vi "flow meter test 2.vi"() -> ()   [LabVIEW 2013]
uses:
  <vilib>/Platform/TimedLoop/XDataNode/timing_clust.ctl
  <vilib>/Platform/TimedLoop/XDataNode/nitl_modes.ctl
  <vilib>/Platform/TimedLoop/XDataNode/wakeup.ctl
  <vilib>/rvi/FXPMathLib/FxpDiv/subVIs/nifxpmath_Div_SimConfig.ctl
  <vilib>/rvi/Emulation/niFpgaSctlEmulationGetInTimedLoop.vi
  <vilib>/rvi/Emulation/niFpgaEmulationReportErrorSimple.vi
  <vilib>/rvi/Emulation/niFpgaGetClockAttributes.vi
  ADC AI Global.vi
  <vilib>/rvi/Emulation/niFpgaProcessEmulError.vi
  ADC AI Global (Avg).vi
  <vilib>/rvi/Emulation/niFpgaCriticalErrorInLSC.vi
  <vilib>/rvi/eio/common/nirviEmuTemplateMethod_errors.vi
  <vilib>/rvi/FXPMathLib/FxpDiv/simVIs/DllFxpDivTemp_sub.vi
  <vilib>/Platform/TimedLoop/XDataNode/XDataNode.xnode
  <vilib>/eio/EIONode/EIONode.xnode
  <vilib>/rvi/FXPMathLib/FxpDiv/XNode/nifxpmath_Div.xnode
  <vilib>/Platform/TimedLoop/XDataNode/XDNodeRunTimeDep.lvlib
panel:
  out "Array 2":fxp<+/-,28,17>[](array[numeric])
  out "Array":fxp<+/-,28,17>[](array[numeric])
  out "Flow":fxp<+/-,28,17>[](array[numeric])
  in  "Freq Flow?":bool
  in  "Max Period (ticks)":u32
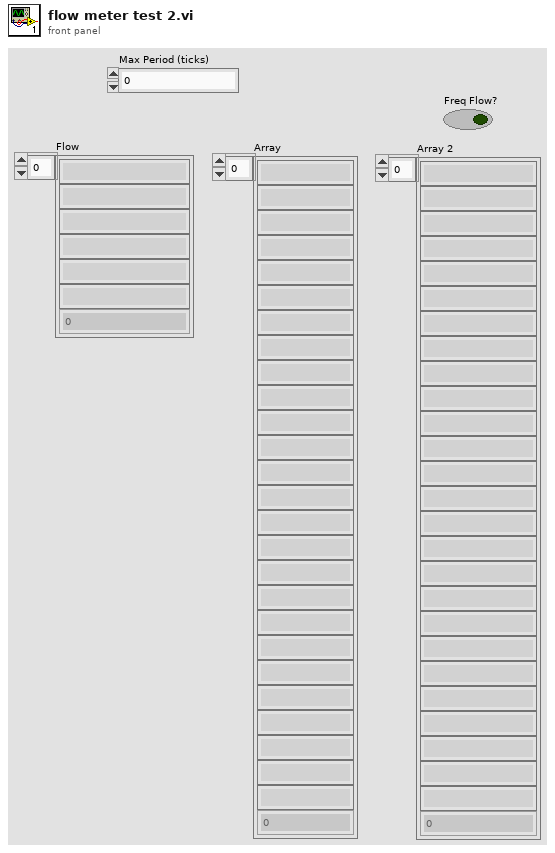
[diagram p1: front panel]
types:
  T1 = typedef "XDNodeRunTimeDep.lvlib/timing_clust.ctl" = cluster{"Expected End [f-1]":u64, "Actual End [f-1]":u64, "Finished Late? [f-1]":bool, "Expected End [i-1]":u64, "Actual End [i-1]":u64, "Finished Late? [i-1]":bool, "Expected Start [i]":u64, "Actual Start [i]":u64, "Expected Start [f]":u64, "Actual Start [f]":u64, "Source Name":string, "Structure Name":string, "Period":i64, "Deadline":i64, "Offset":i64, "Start":i64, "Priority":i32, "Timeout":i32, "Mode":T2, "Wakeup Reason":T3, "Error":errorcluster, "Source Type":string, "Secondary Source Type":string, "Global End Time":u64, "Global Start Time":u64, "Frame Duration":u64, "Iteration Duration":u64, "Assigned CPU":i32, "I/O Scan Engine Mode":u32}
  T2 = typedef "XDNodeRunTimeDep.lvlib/nitl_modes.ctl" = enum32{"No Change", "Process missed periods, maintain original phase", "Discard missed periods, maintain original phase", "Process missed periods, ignore original phase", "Discard missed periods, ignore original phase"}
  T3 = typedef "XDNodeRunTimeDep.lvlib/wakeup.ctl" = enum32{"Normal", "Aborted", "Asynchronous wakeup", "Timing source error", "Timed loop error", "Timeout"}
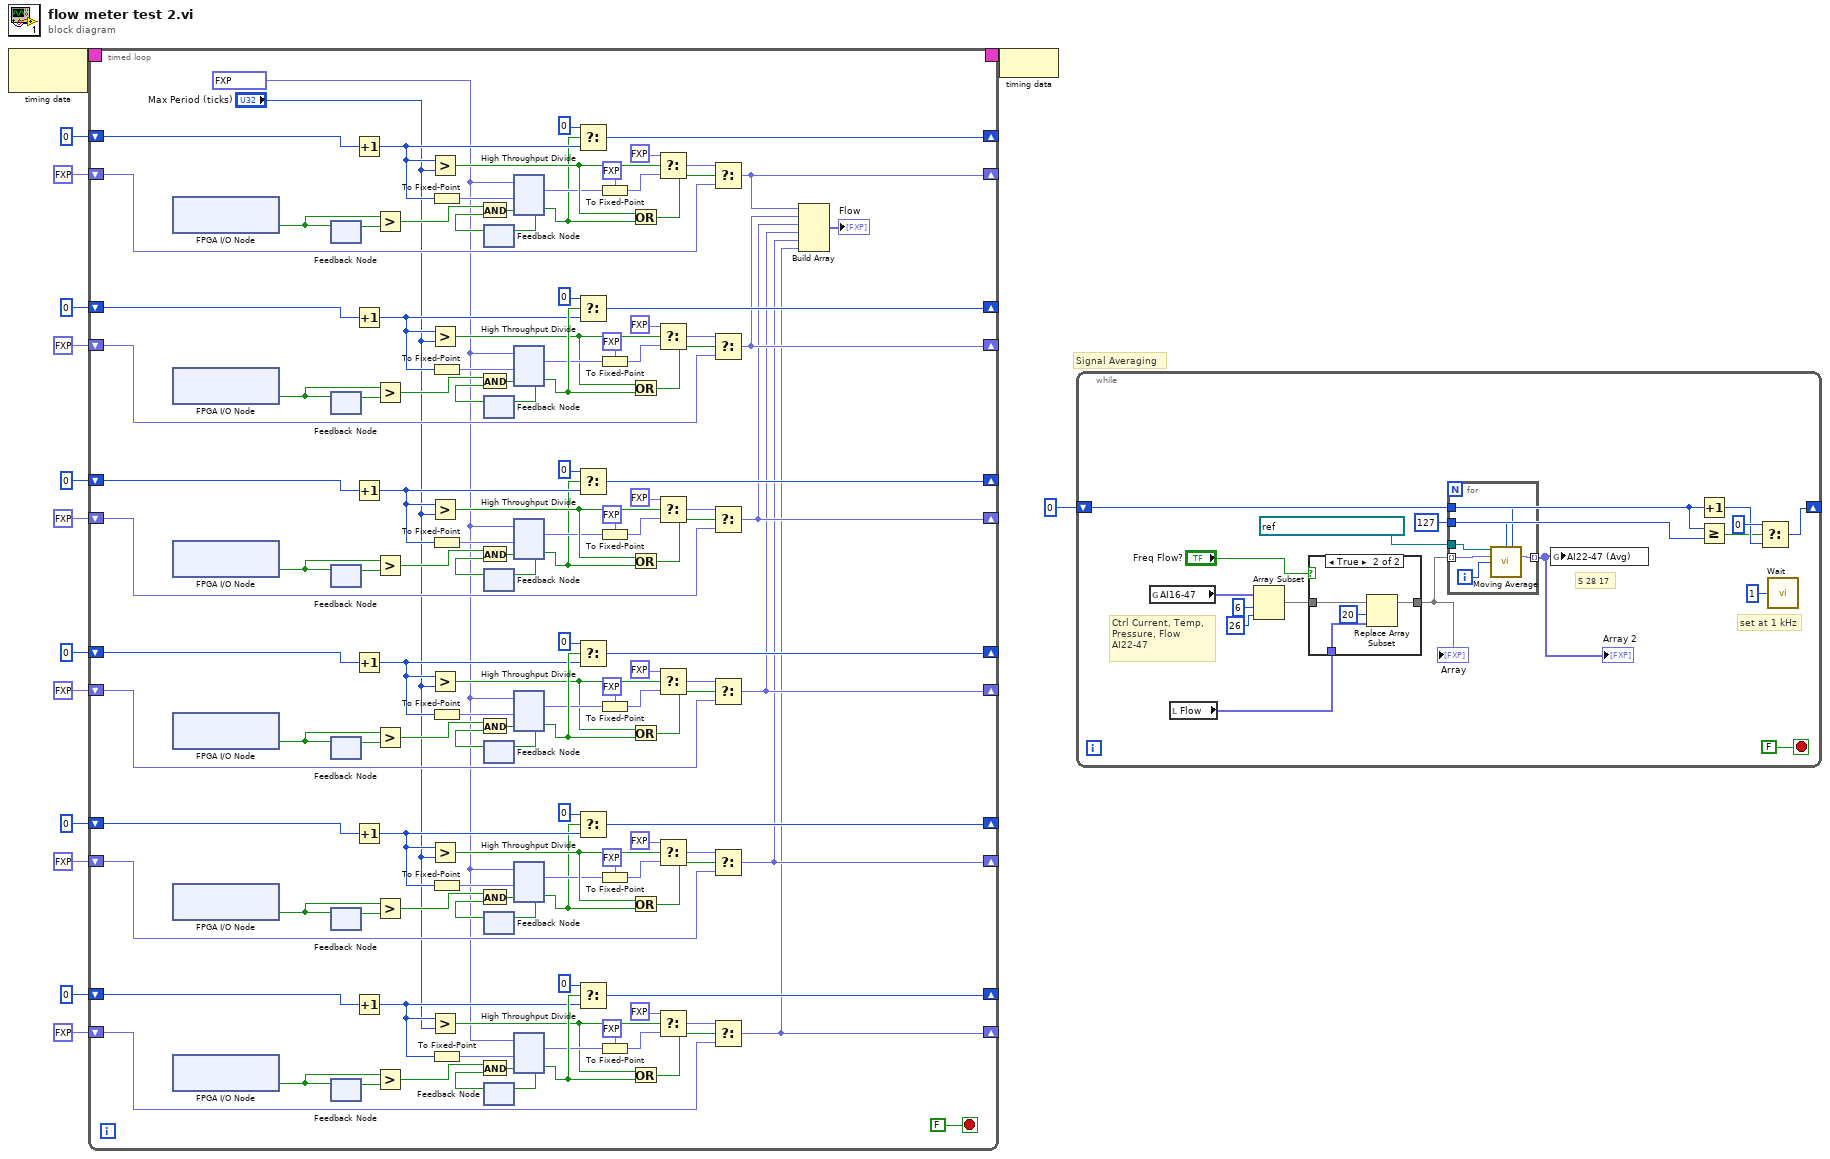
[diagram p0: block diagram]
diagram:
  # "Signal Averaging"
  n1 = node-c288() -> (w15:T1)  [unwired: 1 in]
  n2 = timed-loop {
    timing: w15 -> [_]
    timing-out: [_] -> w14
    shift-right: [w140] -> _
    shift-left: u32 0 ("f") -> [w139]
    shift-right: [w22] -> _
    shift-left: fxp<+/-,28,17> 0.0 ("AI0") -> [w134]
    shift-right: [w109] -> _
    shift-left: u32 0 ("f") -> [w110]
    shift-right: [w21] -> _
    shift-left: fxp<+/-,28,17> 0.0 ("AI0") -> [w115]
    shift-right: [w100] -> _
    shift-left: u32 0 ("f") -> [w99]
    shift-right: [w20] -> _
    shift-left: fxp<+/-,28,17> 0.0 ("AI0") -> [w94]
    shift-right: [w69] -> _
    shift-left: u32 0 ("f") -> [w70]
    shift-right: [w19] -> _
    shift-left: fxp<+/-,28,17> 0.0 ("AI0") -> [w75]
    shift-right: [w60] -> _
    shift-left: u32 0 ("f") -> [w59]
    shift-right: [w18] -> _
    shift-left: fxp<+/-,28,17> 0.0 ("AI0") -> [w54]
    shift-right: [w29] -> _
    shift-left: u32 0 ("f") -> [w30]
    shift-right: [w17] -> _
    shift-left: fxp<+/-,28,17> 0.0 ("AI0") -> [w35]
    stop <- FALSE stop-if-true
    w24 = fxp<+,32,32> 40000000.0 ("x")
    n3 = xnode "FPGA I/O Node"() -> ("RMC/DIO32"=w144:bool)  [unwired: 1 in, 1 out]
    n4 = xnode "FPGA I/O Node"() -> ("RMC/DIO33"=w105:bool)  [unwired: 1 in, 1 out]
    n5 = xnode "FPGA I/O Node"() -> ("RMC/DIO34"=w104:bool)  [unwired: 1 in, 1 out]
    n6 = xnode "FPGA I/O Node"() -> ("RMC/DIO35"=w65:bool)  [unwired: 1 in, 1 out]
    n7 = xnode "FPGA I/O Node"() -> ("RMC/DIO36"=w64:bool)  [unwired: 1 in, 1 out]
    n8 = xnode "FPGA I/O Node"() -> ("RMC/DIO37"=w25:bool)  [unwired: 1 in, 1 out]
    n9 = feedback-in #1(w144) -> ()
    n10 = feedback #1() -> (w143:bool)  [unwired: 1 in]
    n11 = feedback #2() -> (w106:bool)  [unwired: 1 in]
    n12 = feedback-in #2(w105) -> ()
    n13 = feedback #3() -> (w103:bool)  [unwired: 1 in]
    n14 = feedback-in #3(w104) -> ()
    n15 = feedback #4() -> (w66:bool)  [unwired: 1 in]
    n16 = feedback-in #4(w65) -> ()
    n17 = feedback #5() -> (w63:bool)  [unwired: 1 in]
    n18 = feedback-in #5(w64) -> ()
    n19 = feedback #6() -> (w26:bool)  [unwired: 1 in]
    n20 = feedback-in #6(w25) -> ()
    n21 = Increment(x=w139) -> (x+1=w138:u32)
    n22 = Increment(x=w110) -> (x+1=w111:u32)
    n23 = Increment(x=w99) -> (x+1=w98:u32)
    n24 = Increment(x=w70) -> (x+1=w71:u32)
    n25 = Increment(x=w59) -> (x+1=w58:u32)
    n26 = Increment(x=w30) -> (x+1=w31:u32)
    n27 = Greater?(x=w144, y=w143) -> (0:w125:bool)
    n28 = Greater?(x=w105, y=w106) -> (0:w124:bool)
    n29 = Greater?(x=w104, y=w103) -> (0:w85:bool)
    n30 = Greater?(x=w65, y=w66) -> (0:w84:bool)
    n31 = Greater?(x=w64, y=w63) -> (0:w45:bool)
    n32 = Greater?(x=w25, y=w26) -> (0:w44:bool)
    n33 = Greater?(x=w138, y="Max Period (ticks)") -> (0:w142:bool)
    n34 = Greater?(x=w111, y="Max Period (ticks)") -> (0:w107:bool)
    n35 = Greater?(x=w98, y="Max Period (ticks)") -> (0:w102:bool)
    n36 = Greater?(x=w71, y="Max Period (ticks)") -> (0:w67:bool)
    n37 = Greater?(x=w58, y="Max Period (ticks)") -> (0:w62:bool)
    n38 = Greater?(x=w31, y="Max Period (ticks)") -> (0:w27:bool)
    n39 = To Fixed-Point(number=w138) -> (fixed-point=w137:fxp<+,32,32>)  [unwired: 1 in]
    n40 = To Fixed-Point(number=w111) -> (fixed-point=w112:fxp<+,32,32>)  [unwired: 1 in]
    n41 = To Fixed-Point(number=w98) -> (fixed-point=w97:fxp<+,32,32>)  [unwired: 1 in]
    n42 = To Fixed-Point(number=w71) -> (fixed-point=w72:fxp<+,32,32>)  [unwired: 1 in]
    n43 = To Fixed-Point(number=w58) -> (fixed-point=w57:fxp<+,32,32>)  [unwired: 1 in]
    n44 = To Fixed-Point(number=w31) -> (fixed-point=w32:fxp<+,32,32>)  [unwired: 1 in]
    n45 = feedback #7() -> (w126:bool)  [unwired: 1 in]
    n46 = And(x=w125, y=w126) -> (x .and. y?=w127:bool)
    n47 = feedback #8() -> (w123:bool)  [unwired: 1 in]
    n48 = And(x=w124, y=w123) -> (x .and. y?=w122:bool)
    n49 = feedback #9() -> (w86:bool)  [unwired: 1 in]
    n50 = And(x=w85, y=w86) -> (x .and. y?=w87:bool)
    n51 = feedback #10() -> (w83:bool)  [unwired: 1 in]
    n52 = And(x=w84, y=w83) -> (x .and. y?=w82:bool)
    n53 = feedback #11() -> (w46:bool)  [unwired: 1 in]
    n54 = And(x=w45, y=w46) -> (x .and. y?=w47:bool)
    n55 = feedback #12() -> (w43:bool)  [unwired: 1 in]
    n56 = And(x=w44, y=w43) -> (x .and. y?=w42:bool)
    n57 = xnode "High Throughput Divide"("x"=w24, "y"=w137, "input valid"=w127) -> ("x/y"=w133:fxp<+,28,17>, "output valid"=w129:bool, "ready for input"=w128:bool)  [unwired: 1 in]
    n58 = feedback-in #7(w128) -> ()
    n59 = xnode "High Throughput Divide"("x"=w24, "y"=w112, "input valid"=w122) -> ("x/y"=w116:fxp<+,28,17>, "output valid"=w120:bool, "ready for input"=w121:bool)  [unwired: 1 in]
    n60 = feedback-in #8(w121) -> ()
    n61 = xnode "High Throughput Divide"("x"=w24, "y"=w97, "input valid"=w87) -> ("x/y"=w93:fxp<+,28,17>, "output valid"=w89:bool, "ready for input"=w88:bool)  [unwired: 1 in]
    n62 = feedback-in #9(w88) -> ()
    n63 = xnode "High Throughput Divide"("x"=w24, "y"=w72, "input valid"=w82) -> ("x/y"=w76:fxp<+,28,17>, "output valid"=w80:bool, "ready for input"=w81:bool)  [unwired: 1 in]
    n64 = feedback-in #10(w81) -> ()
    n65 = xnode "High Throughput Divide"("x"=w24, "y"=w57, "input valid"=w47) -> ("x/y"=w53:fxp<+,28,17>, "output valid"=w49:bool, "ready for input"=w48:bool)  [unwired: 1 in]
    n66 = feedback-in #11(w48) -> ()
    n67 = xnode "High Throughput Divide"("x"=w24, "y"=w32, "input valid"=w42) -> ("x/y"=w36:fxp<+,28,17>, "output valid"=w40:bool, "ready for input"=w41:bool)  [unwired: 1 in]
    n68 = feedback-in #12(w41) -> ()
    n69 = Select(t=u32 0 ("f"), s=w129, f=w138) -> (s? t:f=w140:u32)
    n70 = Select(t=u32 0 ("f"), s=w120, f=w111) -> (s? t:f=w109:u32)
    n71 = Select(t=u32 0 ("f"), s=w89, f=w98) -> (s? t:f=w100:u32)
    n72 = Select(t=u32 0 ("f"), s=w80, f=w71) -> (s? t:f=w69:u32)
    n73 = Select(t=u32 0 ("f"), s=w49, f=w58) -> (s? t:f=w60:u32)
    n74 = Select(t=u32 0 ("f"), s=w40, f=w31) -> (s? t:f=w29:u32)
    n75 = To Fixed-Point(fixed-point type=fxp<+/-,28,17> 0.0 ("AI0"), number=w133) -> (fixed-point=w131:fxp<+/-,28,17>)
    n76 = To Fixed-Point(fixed-point type=fxp<+/-,28,17> 0.0 ("AI0"), number=w116) -> (fixed-point=w118:fxp<+/-,28,17>)
    n77 = To Fixed-Point(fixed-point type=fxp<+/-,28,17> 0.0 ("AI0"), number=w93) -> (fixed-point=w91:fxp<+/-,28,17>)
    n78 = To Fixed-Point(fixed-point type=fxp<+/-,28,17> 0.0 ("AI0"), number=w76) -> (fixed-point=w78:fxp<+/-,28,17>)
    n79 = To Fixed-Point(fixed-point type=fxp<+/-,28,17> 0.0 ("AI0"), number=w53) -> (fixed-point=w51:fxp<+/-,28,17>)
    n80 = To Fixed-Point(fixed-point type=fxp<+/-,28,17> 0.0 ("AI0"), number=w36) -> (fixed-point=w38:fxp<+/-,28,17>)
    n81 = Or(x=w142, y=w129) -> (x .or. y?=w135:bool)
    n82 = Or(x=w107, y=w120) -> (x .or. y?=w114:bool)
    n83 = Or(x=w102, y=w89) -> (x .or. y?=w95:bool)
    n84 = Or(x=w67, y=w80) -> (x .or. y?=w74:bool)
    n85 = Or(x=w62, y=w49) -> (x .or. y?=w55:bool)
    n86 = Or(x=w27, y=w40) -> (x .or. y?=w34:bool)
    n87 = Select(t=fxp<+/-,28,17> 0.0 ("AI0"), s=w142, f=w131) -> (s? t:f=w136:fxp<+/-,28,17>)
    n88 = Select(t=fxp<+/-,28,17> 0.0 ("AI0"), s=w107, f=w118) -> (s? t:f=w113:fxp<+/-,28,17>)
    n89 = Select(t=fxp<+/-,28,17> 0.0 ("AI0"), s=w102, f=w91) -> (s? t:f=w96:fxp<+/-,28,17>)
    n90 = Select(t=fxp<+/-,28,17> 0.0 ("AI0"), s=w67, f=w78) -> (s? t:f=w73:fxp<+/-,28,17>)
    n91 = Select(t=fxp<+/-,28,17> 0.0 ("AI0"), s=w62, f=w51) -> (s? t:f=w56:fxp<+/-,28,17>)
    n92 = Select(t=fxp<+/-,28,17> 0.0 ("AI0"), s=w27, f=w38) -> (s? t:f=w33:fxp<+/-,28,17>)
    n93 = Select(t=w136, s=w135, f=w134) -> (s? t:f=w22:fxp<+/-,28,17>)
    n94 = Select(t=w113, s=w114, f=w115) -> (s? t:f=w21:fxp<+/-,28,17>)
    n95 = Select(t=w96, s=w95, f=w94) -> (s? t:f=w20:fxp<+/-,28,17>)
    n96 = Select(t=w73, s=w74, f=w75) -> (s? t:f=w19:fxp<+/-,28,17>)
    n97 = Select(t=w56, s=w55, f=w54) -> (s? t:f=w18:fxp<+/-,28,17>)
    n98 = Select(t=w33, s=w34, f=w35) -> (s? t:f=w17:fxp<+/-,28,17>)
    n99 = Build Array(w22, w21, w20, w19, w18, w17) -> (→"Flow":fxp<+/-,28,17>[])
  }
  n100 = node-c288(w14) -> ()
  n101 = while {
    shift-right: [w332] -> _
    shift-left: 0 ("Moving Point Index") -> [w333]
    stop <- FALSE stop-if-true
    w331 = 127 ("N (# of Ave Pts 8 max)")
    # "Ctrl Current, Temp,\nPressure, Flow\nAI22-47"
    # "S 28 17"
    # "set at 1 kHz"
    n102 = global read "ADC AI Global.vi" "AI16-47"() -> (w327:fxp<+/-,28,17>[])
    n103 = local read "Flow"() -> (w322:fxp<+/-,28,17>[])
    n104 = Array Subset(array=w327, index=6, length=26) -> (w324:fxp<+/-,28,17>[])
    n105 = case shown="True" "Freq Flow?" {
      tunnel: w324 -> [w339 w343]
      tunnel: w322 -> [_ w342]
      tunnel: [w339 w340] -> w323
      frame False {
      }
      frame True {
        n106 = Replace Array Subset(array=w343, new element=w342, index=20) -> (w340:fxp<+/-,28,17>[])
      }
    }
    "Array" <- w323
    n107 = for {
      tunnel: w333 -> [w344]
      tunnel: w331 -> [w345]
      tunnel: [w349] -> w326 mode=indexing
      tunnel: w323 -> [w348] mode=indexing
      tunnel: refnum<k21> "Running Avg Memory" ("Memory") -> [w347]
      i -> [w346]
      n108 = call "Moving Average.vi"("Memory In"=w347, "N (# of Ave Pts 127 max)"=w345, "Moving Point Index"=w344, "Data IN"=w348, "Channel#"=w346) -> ("Averaged Data"=w349:fxp<+/-,28,17>)  [unwired: 10 in]
    }
    "Array 2" <- w326
    n109 = global write "ADC AI Global (Avg).vi" "AI22-47 (Avg)"(w326) -> ()
    n110 = Increment(x=w333) -> (x+1=w335:i32)
    n111 = Greater Or Equal?(x=w333, y=w331) -> (x >= y?=w334:bool)
    n112 = Select(t=0, s=w334, f=w335) -> (s? t:f=w332:i32)
    n113 = call "Wait"("Count(mSec)"=u32 1) -> ()  [unwired: 1 out]
  }
